vi "Create.vi"(8 "error in (no error)":errorcluster, 9 "RemoteDataService":refnum<class "RemoteDataService.lvclass">, 10 "ChannelService":refnum<class "ChannelService.lvclass">) -> (0 "error out":errorcluster, 3 "TelemetryAPI out":refnum<class "TelemetryAPI.lvclass">)   [LabVIEW 2020, in "Volatus.lvlib" / "TelemetryAPI.lvclass"]
uses:
  TelemetryAPI.lvclass
  TelemetryAPI.lvclass/TelemetryAPI.ctl
  lv-vecto/Vecto/ChannelService/ChannelService.lvclass
  lv-vecto/Vecto/RemoteDataService/RemoteDataService.lvclass
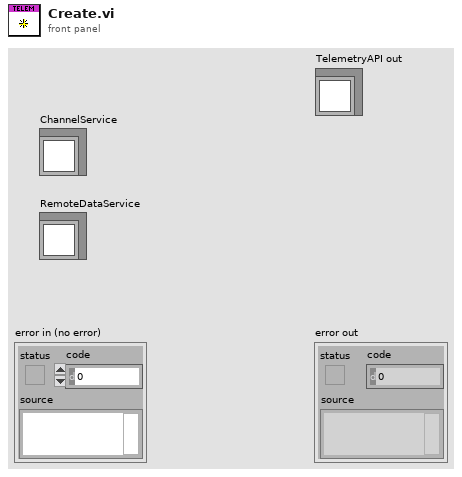
[diagram p1: front panel]
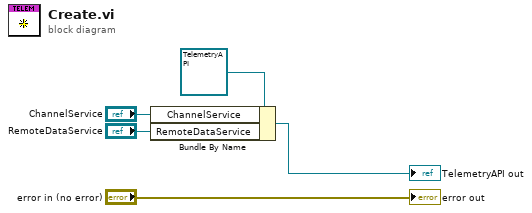
[diagram p0: block diagram]
diagram:
  n1 = Bundle By Name(cluster=refnum<class "TelemetryAPI.lvclass"> refnum ("TelemetryAPI in"), "ChannelService"="ChannelService", "RemoteDataService"="RemoteDataService") -> (→"TelemetryAPI out":refnum<class "TelemetryAPI.lvclass">)
  "error out" <- "error in (no error)"
